vi "SetPitch.vi"(8 "error in (no error)":errorcluster, 9 "speed in mm/s":dbl=1.0, 10 "axis":i32, 11 "DLOwis in":refnum<class "DLOwis.lvclass">) -> (0 "error out":errorcluster, 3 "DLOwis out":refnum<class "DLOwis.lvclass">)   [LabVIEW 2020, in "DLOwis.lvclass"]
uses:
  DLOwis.lvclass
  C:/dev/TRANCON/Classes/Delay Line/DelayLine.lvclass
  DelayLine.lvclass/DelayLine.ctl
  DelayLine.lvclass
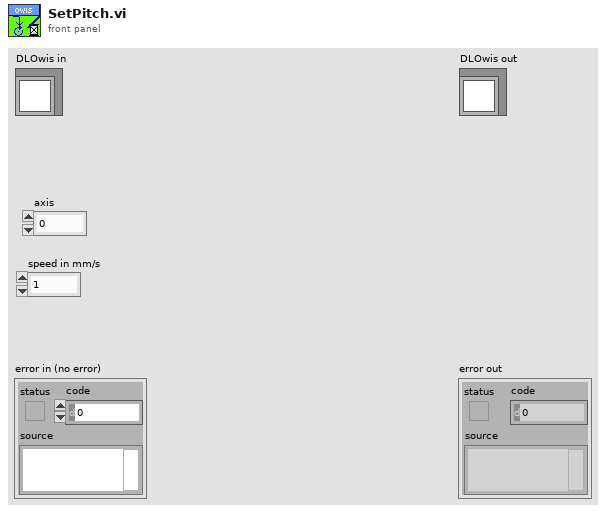
[diagram p1: front panel]
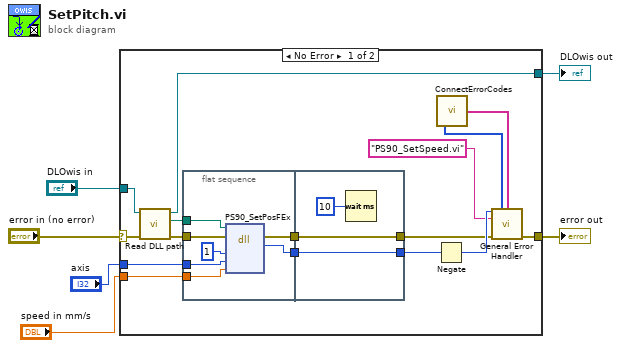
[diagram p0: block diagram]
diagram:
  n1 = case shown="No Error" "error in (no error)" {
    selector: "error in (no error)" -> [w19 w33]
    tunnel: [w22 w33] -> w5
    tunnel: "DLOwis in" -> [w21 w34]
    tunnel: [w20 w34] -> w6
    tunnel: "speed in mm/s" -> [w12 _]
    tunnel: "axis" -> [w11 _]
    frame No Error {
      n2 = call "Read DLL path.vi"("error in (no error)"=w19, "DelayLine in"=w21) -> ("error out"=w14:errorcluster, "DLL path"=w13:path, "DelayLine out"=w20:refnum<class "DLOwis.lvclass">)  [unwired: 7 in]
      n3 = flat-sequence {
        tunnel: w14 -> [w26]
        tunnel: w13 -> [w23]
        tunnel: w12 -> [w27]
        tunnel: w11 -> [w28]
        tunnel: [w25] -> w9
        tunnel: [w24] -> w8
        tunnel: [w31] -> w10
        tunnel: w9 -> [w31]
        tunnel: w8 -> [w30]
        tunnel: [w30] -> w7
        frame #0 {
          n4 = dll-call lib="C:/Dev/TRANCON/DLL/ps90.dll" fn="PS90_SetPosFEx" label="PS90_Set\nPosFEx"(path in=w23, error in=w26, "Index"=1, "AxisNr"=w28, "dValue"=w27) -> (error out=w25:errorcluster, "Rückgabetyp"=w24:i32)  [unwired: 4 in, 1 out]
        }
        frame #1 {
          n5 = Wait (ms)(milliseconds to wait=u32 10) -> ()  [unwired: 1 out]
        }
      }
      n6 = Negate(x=w7) -> (-x=w18:i32)
      n7 = call "ConnectErrorCodes.vi"() -> ("[user-defined descriptions]"=w15:string[], "[user-defined codes]"=w16:i32[])
      n8 = call <vilib>:"General Error Handler.vi"("[error code] (0)"=w18, "[user-defined codes]"=w16, "[user-defined descriptions]"=w15, "[error source] (\" \")"="PS90_SetSpeed.vi", "error in (no error)"=w10) -> ("error out"=w22:errorcluster)  [unwired: 6 in, 4 out]
    }
    frame Error {
    }
  }
  "error out" <- w5
  "DLOwis out" <- w6
